vi "Profile Test Program.vi"() -> ()   [LabVIEW 2017]
uses:
  <vilib>/Utility/file.llb/Read Delimited Spreadsheet (DBL).vi
  <vilib>/Utility/file.llb/Write Delimited Spreadsheet (DBL).vi
panel:
  out "error out 2":errorcluster
  out "error out":errorcluster
  in  "Profile Name":string="Profile1"
  in  "Load":bool
  in  "Save":bool
  in  "High Gear Turning Multiplier":dbl=0.65 format="%#_13g"
  in  "Turning Sensitity":dbl=0.4 format="%#_13g"
  in  "Foreward Sensitivity":dbl=1.0 format="%#_13g"
  in  "Max Speed":dbl=1.0 format="%#_13g"
  in  "Autoshift":bool=TRUE
  in  "Direction Toggle":bool=TRUE
  in  "High Gear":bool=TRUE
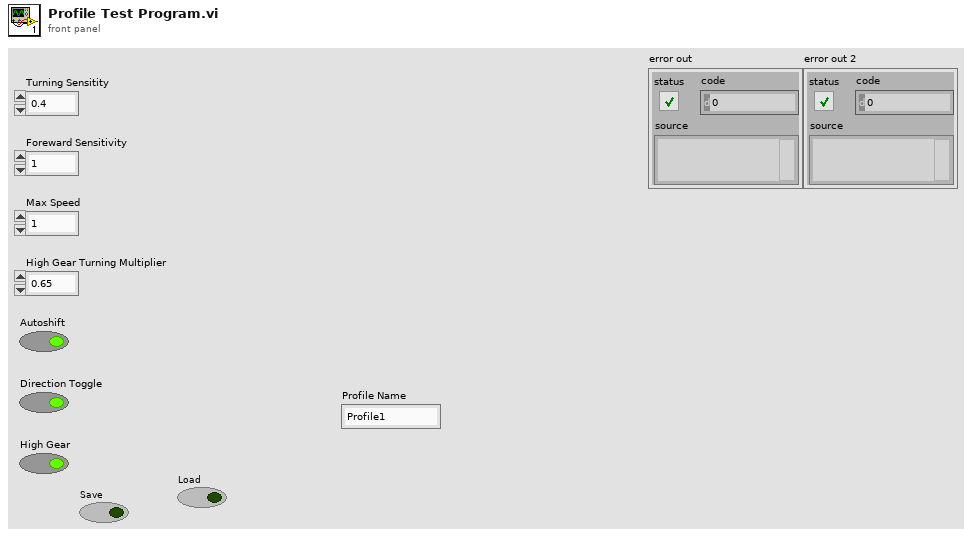
[diagram p1: front panel]
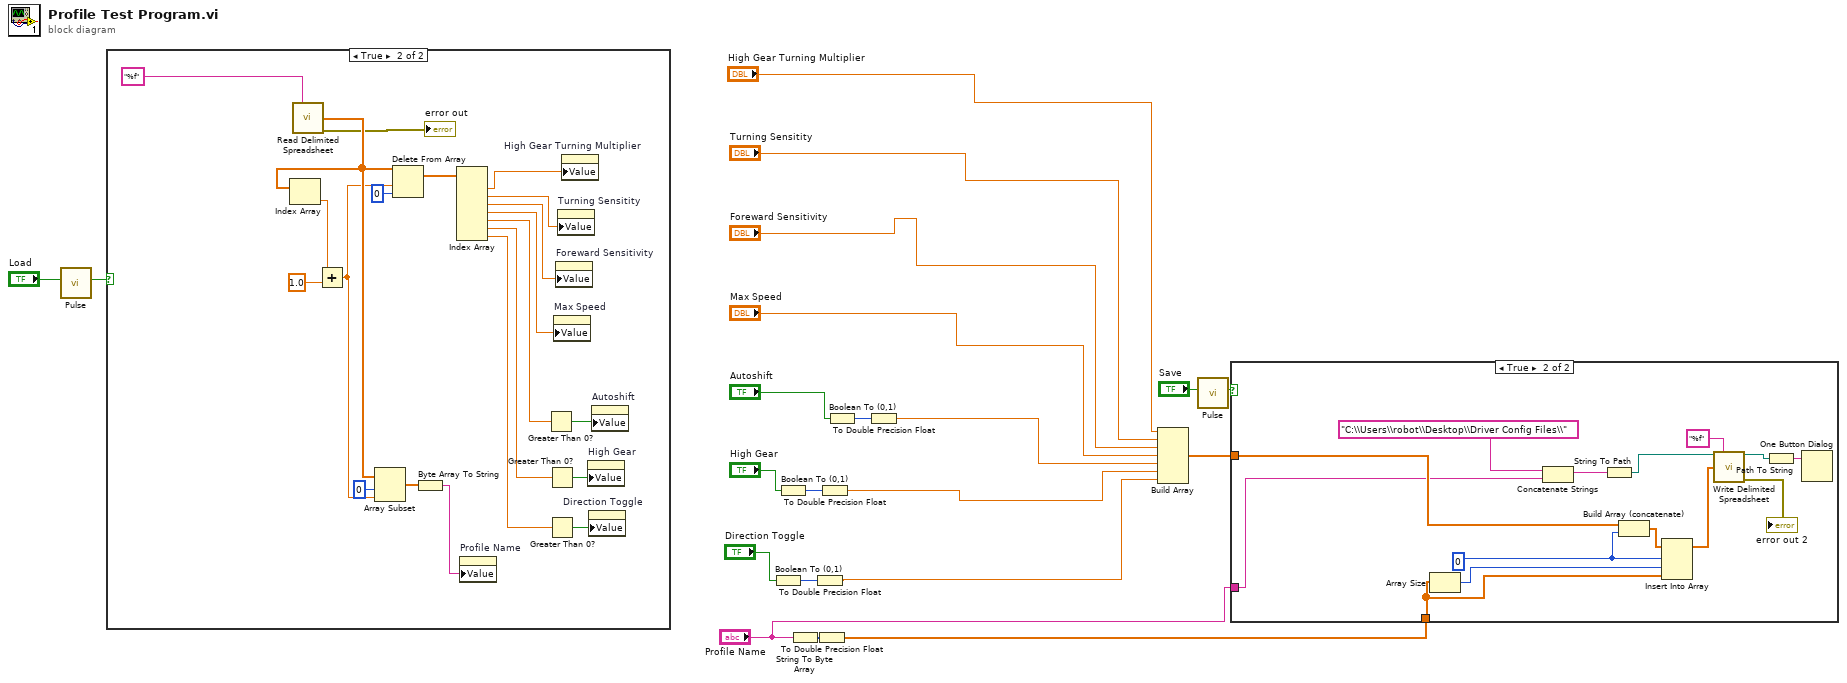
[diagram p0: block diagram]
diagram:
  n1 = call "Pulse.vi"("Input"="Load") -> ("Output"=w5:bool)  [unwired: 10 in]
  n2 = case shown="True" w5 {
    frame False {
    }
    frame True {
      n3 = call-poly <vilib>:"Read Delimited Spreadsheet.vi"("format (%.3f)"="%f") -> ("first row"=w39:dbl[], "error out"=→"error out":errorcluster)  [unwired: 9 in, 4 out]
      n4 = Index Array(array=w39) -> (element=w24:dbl)  [unwired: 1 in]
      n5 = Add(x=w24, y=1.0) -> (x+y=w23:dbl)
      n6 = Array Subset(array=w39, index=0, length=w23) -> (w40:dbl[])
      n7 = Delete From Array(array=w39, length=w23, index=0) -> (array with subset deleted=w37:dbl[])  [unwired: 1 out]
      n8 = Byte Array To String(unsigned byte array=w40) -> (string=w26:string)
      n9 = Index Array(array=w37) -> (element #1=w36:dbl, element #2=w35:dbl, element #3=w34:dbl, element #4=w33:dbl, element #5=w32:dbl, element #6=w31:dbl, element #7=w30:dbl)  [unwired: 7 in]
      n10 = property on="Profile Name" class="Str"("Value"=w26) -> ()  [unwired: 2 in, 2 out]
      n11 = Greater Than 0?(x=w32) -> (x > 0?=w27:bool)
      n12 = Greater Than 0?(x=w31) -> (x > 0?=w28:bool)
      n13 = Greater Than 0?(x=w30) -> (x > 0?=w29:bool)
      n14 = property on="Max Speed" class="DigNum (strict)"("Value"=w33) -> ()  [unwired: 2 in, 2 out]
      n15 = property on="Foreward Sensitivity" class="DigNum (strict)"("Value"=w34) -> ()  [unwired: 2 in, 2 out]
      n16 = property on="Turning Sensitity" class="DigNum (strict)"("Value"=w35) -> ()  [unwired: 2 in, 2 out]
      n17 = property on="High Gear Turning Multiplier" class="DigNum (strict)"("Value"=w36) -> ()  [unwired: 2 in, 2 out]
      n18 = property on="High Gear" class="Bool (strict)"("Value"=w28) -> ()  [unwired: 2 in, 2 out]
      n19 = property on="Direction Toggle" class="Bool (strict)"("Value"=w29) -> ()  [unwired: 2 in, 2 out]
      n20 = property on="Autoshift" class="Bool (strict)"("Value"=w27) -> ()  [unwired: 2 in, 2 out]
    }
  }
  n21 = Boolean To (0,1)(Boolean="Direction Toggle") -> (0, 1=w9:i16)
  n22 = Boolean To (0,1)(Boolean="High Gear") -> (0, 1=w12:i16)
  n23 = String To Byte Array(string="Profile Name") -> (unsigned byte array=w4:u8[])
  n24 = To Double Precision Float(number=w9) -> (double precision float=w8:dbl)
  n25 = To Double Precision Float(number=w4) -> (double precision float=w2:dbl[])
  n26 = To Double Precision Float(number=w12) -> (double precision float=w10:dbl)
  n27 = Boolean To (0,1)(Boolean="Autoshift") -> (0, 1=w14:i16)
  n28 = To Double Precision Float(number=w14) -> (double precision float=w13:dbl)
  n29 = Build Array("High Gear Turning Multiplier", "Turning Sensitity", "Foreward Sensitivity", "Max Speed", w13, w10, w8) -> (w3:dbl[])
  n30 = call "Pulse.vi"("Input"="Save") -> ("Output"=w16:bool)  [unwired: 10 in]
  n31 = case shown="True" w16 {
    tunnel: w3 -> [_ w52]
    tunnel: w2 -> [_ w54]
    tunnel: "Profile Name" -> [_ w48]
    frame False {
    }
    frame True {
      w51 = 0 ("index")
      n32 = Array Size(array=w54) -> (size(s)=w55:i32)
      n33 = Concatenate Strings("C:\\Users\\robot\\Desktop\\Driver Config Files\\" ("string"), w48) -> (w47:string)
      n34 = String To Path(string=w47) -> (path=w46:path)
      n35 = Build Array (concatenate)(w52, w51) -> (w50:dbl[])
      n36 = Insert Into Array(array=w50, index=w51, new element #1=w55, new element #2=w54) -> (w53:dbl[])
      n37 = call-poly <vilib>:"Write Delimited Spreadsheet.vi"("file path (dialog if empty)"=w46, "format (%.3f)"="%f", "1D data"=w53) -> ("new file path (Not A Path if cancelled)"=w44:path, "error out"=→"error out 2":errorcluster)  [unwired: 11 in]
      n38 = Path To String(path=w44) -> (string=w45:string)
      n39 = One Button Dialog(message=w45) -> ()  [unwired: 1 in, 1 out]
    }
  }
